vi "PIDMotor.vi"(0 "Motor Object":T5, 1 "Robot Configuration":T1={"wheel parameters"={"wheel radius"=0.05, "gear ratio"=1.0, "forward rotation direction"=0}, "wheel separation"=0.19, "Encoder Pulse Per Rev"=1856.0, "Update Period (sec)"=0.02, "Initial posture frame"=[0.0, 0.0, 0.0]} {"wheel parameters"."forward rotation direction" items=["Clockwise", "Counterclockwise"]}, 2 "calculated wheel states":T18[](array[typedef]), 3 "Wheel Velocity":T19) -> ()   [LabVIEW 2016]
uses:
  <vilib>/robotics/Steering/Wheel/Wheel State.ctl
  MotorObject.ctl
  <vilib>/myRIO/Instrument Drivers/Onboard IO/PWM/typedefs/PWM Reference.ctl
  <vilib>/myRIO/Common/Instrument Driver Framework/Utilities/typedefs/myRIO Generic Hardware Reference.ctl
  <vilib>/myRIO/Common/Instrument Driver Framework/Utilities/typedefs/Hardware Version Enum.ctl
  <vilib>/myRIO/Common/Instrument Driver Framework/Utilities/typedefs/myRIO v1.0 Reference.ctl
  <vilib>/myRIO/Common/Instrument Driver Framework/Utilities/typedefs/Generic FPGA Reference.ctl
  <vilib>/myRIO/Common/Instrument Driver Framework/myRIO v1.0/PWM/typedefs/PWM Channels Enum.ctl
  <vilib>/myRIO/Instrument Drivers/Onboard IO/PWM/typedefs/PWM Configuration.ctl
  <vilib>/myRIO/Instrument Drivers/Onboard IO/DIO/typedefs/DIO Reference.ctl
  <vilib>/myRIO/Common/Instrument Driver Framework/myRIO v1.0/DIO/typedefs/DIO Channels List.ctl
  <vilib>/myRIO/Common/Instrument Driver Framework/myRIO v1.0/DIO/typedefs/DIO Channels Enum.ctl
  <vilib>/myRIO/Instrument Drivers/Onboard IO/Encoder/typedefs/Encoder Reference.ctl
  <vilib>/myRIO/Common/Instrument Driver Framework/myRIO v1.0/Encoder/typedefs/Encoder Channels Enum.ctl
  Configurations.ctl
  <vilib>/robotics/Steering/Wheel/Wheel Parameters.ctl
  <vilib>/robotics/Steering/Wheel/Rotation Direction.ctl
  <vilib>/myRIO/Instrument Drivers/Onboard IO/PWM/vis/Set Duty Cycle and Frequency.vi
  <vilib>/myRIO/Common/Instrument Driver Framework/myRIO v1.0/DIO/vis/myRIO v1.0 Write DIO.vi
  <vilib>/myRIO/Common/Instrument Driver Framework/roboRIO v1.0/DIO/vis/roboRIO v1.0 Write DIO.vi
  <vilib>/Utility/error.llb/Error Cluster From Error Code.vi
  <vilib>/addons/control/pid/pid.llb/PID (DBL).vi
  <vilib>/myRIO/Common/Instrument Driver Framework/myRIO v1.0/PWM/vis/myRIO v1.0 Write PWM.vi
  <vilib>/myRIO/Common/Instrument Driver Framework/roboRIO v1.0/PWM/vis/roboRIO v1.0 Write PWM.vi
  <vilib>/addons/control/pid/NI_PID_pid.lvlib
  <vilib>/myRIO/Instrument Drivers/Onboard IO/PWM/PWM.lvlib
  <vilib>/myRIO/Instrument Drivers/Onboard IO/DIO/DIO.lvlib
  <vilib>/robotics/Steering/Wheel/NI_Robotics_Wheel.lvclass
  <vilib>/myRIO/Instrument Drivers/Onboard IO/Encoder/Encoder.lvlib
panel:
  out "DIR Right":bool
  in  "PID gains Motor Right":T4={"proportional gain (Kc)"=4.8, "integral time (Ti, min)"=0.01, "derivative time (Td, min)"=0.001} {"derivative time (Td, min)" format="%.3f"; "integral time (Ti, min)" format="%.3f"; "proportional gain (Kc)" format="%.3f"}
  out "PWM Signal Right":dbl
  out "PWM Signal Left":dbl
  in  "PID gains Motor Left":T4={"proportional gain (Kc)"=5.1, "integral time (Ti, min)"=0.01, "derivative time (Td, min)"=0.001} {"derivative time (Td, min)" format="%.3f"; "integral time (Ti, min)" format="%.3f"; "proportional gain (Kc)" format="%.3f"}
  out "DIR Left":bool
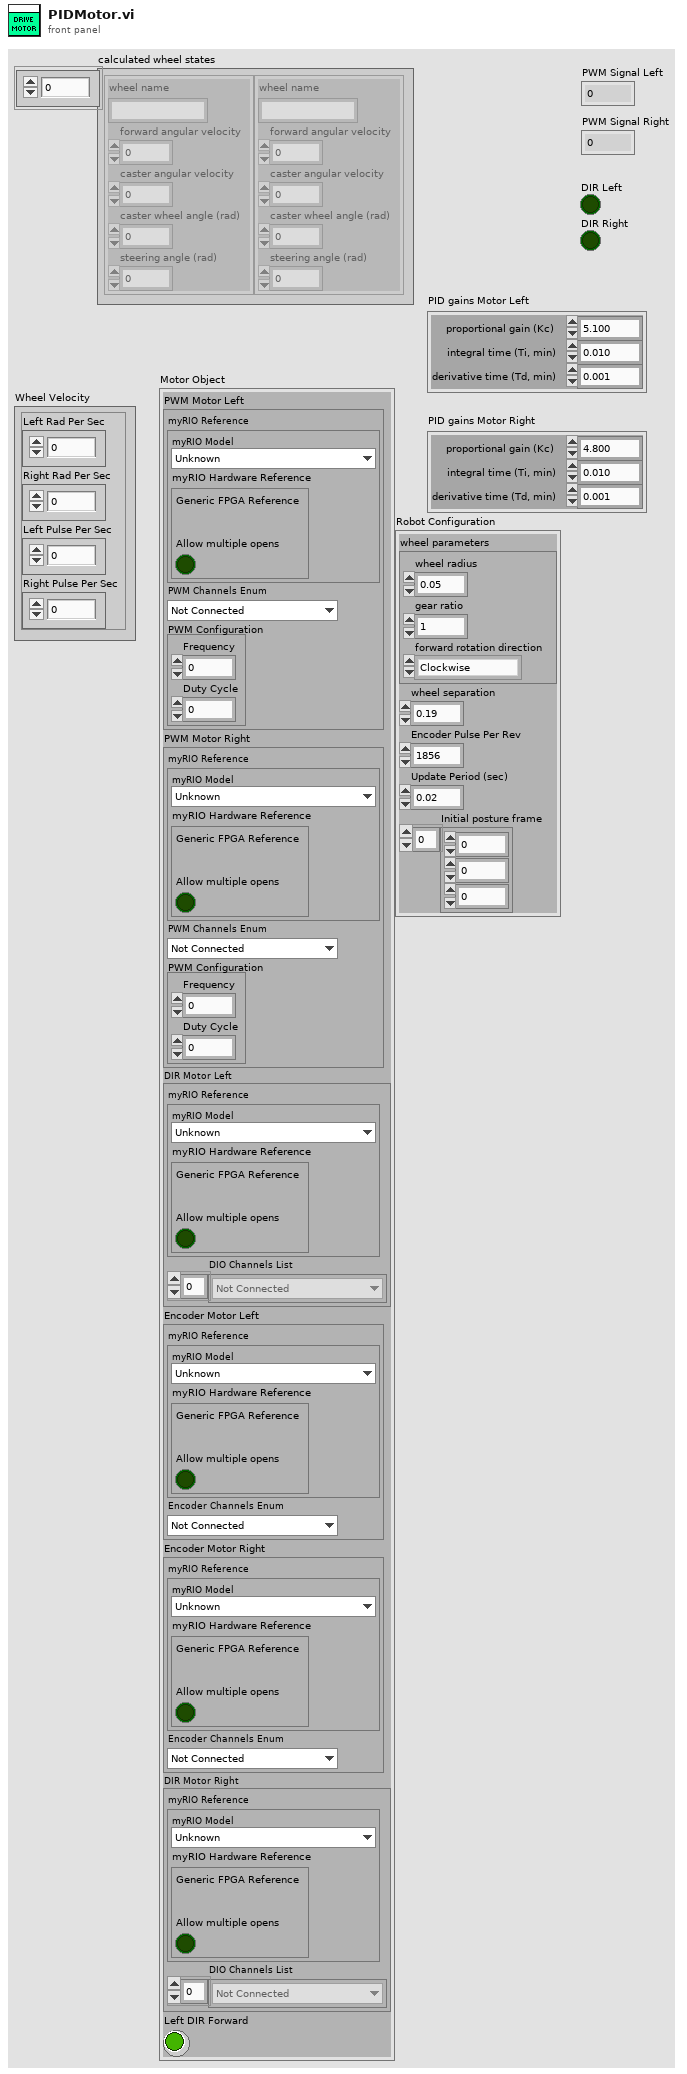
[diagram p1: front panel]
types:
  T1 = typedef "Configurations.ctl" = cluster{"wheel parameters":T2, "wheel separation":dbl, "Encoder Pulse Per Rev":dbl, "Update Period (sec)":dbl, "Initial posture frame":dbl[]}
  T2 = typedef "NI_Robotics_Wheel.lvclass/Wheel Parameters.ctl" = cluster{"wheel radius":dbl, "gear ratio":dbl, "forward rotation direction":T3}
  T3 = typedef "NI_Robotics_Wheel.lvclass/Rotation Direction.ctl" = u16
  T4 = cluster{"proportional gain (Kc)":dbl, "integral time (Ti, min)":dbl, "derivative time (Td, min)":dbl}
  T5 = typedef "MotorObject.ctl" = cluster{"PWM Motor Left":T6, "PWM Motor Right":T6, "DIR Motor Left":T13, "Encoder Motor Left":T16, "Encoder Motor Right":T16, "DIR Motor Right":T13, "Left DIR Forward":bool}
  T6 = typedef "PWM.lvlib/PWM Reference.ctl" = cluster{"myRIO Reference":T7, "PWM Channels Enum":T11, "PWM Configuration":T12}
  T7 = typedef "myRIO Generic Hardware Reference.ctl" = cluster{"myRIO Model":T8, "myRIO Hardware Reference":T9}
  T8 = typedef "Hardware Version Enum.ctl" = enum16{"Unknown", "myRIO-1900", "myRIO-1950", "roboRIO", "NI ELVIS RIO CM"}
  T9 = typedef "myRIO v1.0 Reference.ctl" = cluster{"Generic FPGA Reference":T10, "Allow multiple opens":bool}
  T10 = typedef "Generic FPGA Reference.ctl" = refnum<k20>
  T11 = typedef "PWM Channels Enum.ctl" = enum16{"Not Connected", "C/PWM0", "C/PWM1", "A/PWM0", "A/PWM1", "A/PWM2", "B/PWM0", "B/PWM1", "B/PWM2", "PWM/PWM0", "PWM/PWM1", "PWM/PWM2", "PWM/PWM3", "PWM/PWM4", "PWM/PWM5", "PWM/PWM6", "PWM/PWM7", "PWM/PWM8", "PWM/PWM9"}
  T12 = typedef "PWM.lvlib/PWM Configuration.ctl" = cluster{"Frequency":dbl, "Duty Cycle":dbl}
  T13 = typedef "DIO.lvlib/DIO Reference.ctl" = cluster{"myRIO Reference":T7, "DIO Channels List":T14}
  T14 = typedef "DIO Channels List.ctl" = T15[]
  T15 = typedef "DIO Channels Enum.ctl" = enum16{"Not Connected", "C/DIO0", "C/DIO1", "C/DIO2", "C/DIO3", "C/DIO4", "C/DIO5", "C/DIO6", "C/DIO7", "A/DIO0", "A/DIO1", "A/DIO2", "A/DIO3", "A/DIO4", "A/DIO5", "A/DIO6", "A/DIO7", "A/DIO8", "A/DIO9", "A/DIO10", "A/DIO11", "A/DIO12", "A/DIO13", "A/DIO14", "A/DIO15", "B/DIO0", "B/DIO1", "B/DIO2", "B/DIO3", "B/DIO4", "B/DIO5", "B/DIO6", "B/DIO7", "B/DIO8", "B/DIO9", "B/DIO10", "B/DIO11", "B/DIO12", "B/DIO13", "B/DIO14", "B/DIO15", "LED0", "LED1", "LED2", "LED3", "Button0", "DIO/DIO0", "DIO/DIO1", "DIO/DIO2", "DIO/DIO3", "DIO/DIO4", "DIO/DIO5", "DIO/DIO6", "DIO/DIO7", "DIO/DIO8", "DIO/DIO9", "SPI/CS0", "SPI/CS1", "SPI/CS2", "SPI/CS3", "LED RADIO (Green)", "LED RADIO (Red)", "LED COMM (Green)", "LED COMM (Red)", "LED MODE (Green)", "LED MODE (Red)"}
  T16 = typedef "Encoder.lvlib/Encoder Reference.ctl" = cluster{"myRIO Reference":T7, "Encoder Channels Enum":T17}
  T17 = typedef "Encoder Channels Enum.ctl" = enum16{"Not Connected", "C/ENC0", "C/ENC1", "A/ENC", "B/ENC", "DIO/ENC0", "DIO/ENC1", "DIO/ENC2", "DIO/ENC3", "DIO/ENC4"}
  T18 = typedef "NI_Robotics_Wheel.lvclass/Wheel State.ctl" = cluster{"wheel name":string, "forward angular velocity":dbl, "caster angular velocity":dbl, "caster wheel angle (rad)":dbl, "steering angle (rad)":dbl}
  T19 = cluster{"Left Rad Per Sec":dbl, "Right Rad Per Sec":dbl, "Left Pulse Per Sec":dbl, "Right Pulse Per Sec":dbl}
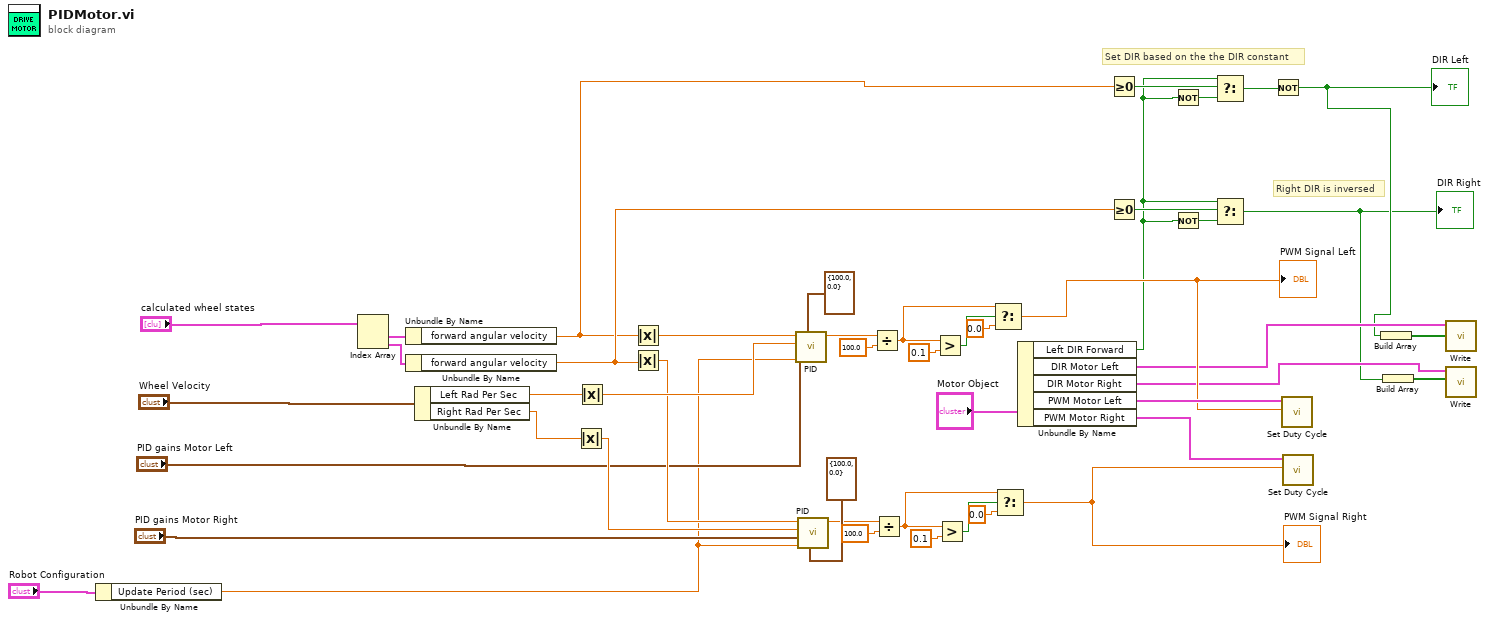
[diagram p0: block diagram]
diagram:
  # "Right DIR is inversed"
  # "Set DIR based on the the DIR constant"
  n1 = Unbundle By Name("Robot Configuration") -> ("Update Period (sec)"=w1:dbl)
  n2 = Index Array(array="calculated wheel states") -> (element #1=w36:T18, element #2=w37:T18)  [unwired: 2 in]
  n3 = Unbundle By Name(w36) -> ("forward angular velocity"=w5:dbl)
  n4 = Unbundle By Name(w37) -> ("forward angular velocity"=w6:dbl)
  n5 = Unbundle By Name("Wheel Velocity") -> ("Left Rad Per Sec"=w39:dbl, "Right Rad Per Sec"=w26:dbl)
  n6 = Absolute Value(x=w26) -> (abs(x)=w24:dbl)
  n7 = Absolute Value(x=w39) -> (abs(x)=w40:dbl)
  n8 = Absolute Value(x=w5) -> (abs(x)=w27:dbl)
  n9 = Absolute Value(x=w6) -> (abs(x)=w25:dbl)
  n10 = call-poly <vilib>:"PID.vi"("output range"=cluster{"output high":dbl, "output low":dbl} {"output high"=100.0, "output low"=0.0}, "dt (s)"=w1, "PID gains"="PID gains Motor Left", "process variable"=w40, "setpoint"=w27) -> ("output"=w47:dbl)  [unwired: 5 in, 1 out]
  n11 = call-poly <vilib>:"PID.vi"("output range"=cluster{"output high":dbl, "output low":dbl} {"output high"=100.0, "output low"=0.0}, "dt (s)"=w1, "PID gains"="PID gains Motor Right", "process variable"=w24, "setpoint"=w25) -> ("output"=w28:dbl)  [unwired: 5 in, 1 out]
  n12 = Divide(x=w47, y=100.0) -> (x/y=w45:dbl)
  n13 = Divide(x=w28, y=100.0) -> (x/y=w30:dbl)
  n14 = Greater?(x=w45, y=0.1) -> (0:w44:bool)
  n15 = Greater?(x=w30, y=0.1) -> (0:w31:bool)
  n16 = Select(t=w45, s=w44, f=0.0) -> (s? t:f=w19:dbl)
  "PWM Signal Left" <- w19
  n17 = Select(t=w30, s=w31, f=0.0) -> (s? t:f=w18:dbl)
  "PWM Signal Right" <- w18
  n18 = Unbundle By Name("Motor Object") -> ("Left DIR Forward"=w13:bool, "DIR Motor Left"=w12:T13, "DIR Motor Right"=w11:T13, "PWM Motor Left"=w21:T6, "PWM Motor Right"=w20:T6)
  n19 = Greater Or Equal To 0?(x=w5) -> (x >= 0?=w14:bool)
  n20 = Greater Or Equal To 0?(x=w6) -> (x >= 0?=w17:bool)
  n21 = Not(x=w13) -> (.not. x?=w15:bool)
  n22 = Not(x=w13) -> (.not. x?=w16:bool)
  n23 = Select(t=w13, s=w14, f=w15) -> (s? t:f=w10:bool)
  n24 = Select(t=w13, s=w17, f=w16) -> (s? t:f=w3:bool)
  "DIR Right" <- w3
  n25 = Not(x=w10) -> (.not. x?=w4:bool)
  "DIR Left" <- w4
  n26 = call <vilib>:"Set Duty Cycle.vi"("Duty Cycle"=w19, "PWM Ref In"=w21) -> ()  [unwired: 7 in, 2 out]
  n27 = call <vilib>:"Set Duty Cycle.vi"("Duty Cycle"=w18, "PWM Ref In"=w20) -> ()  [unwired: 7 in, 2 out]
  n28 = Build Array(w4) -> (w9:bool[])
  n29 = Build Array(w3) -> (w8:bool[])
  n30 = call <vilib>:"Write.vi"("Values"=w9, "DIO Ref In"=w12) -> ()  [unwired: 7 in, 2 out]
  n31 = call <vilib>:"Write.vi"("Values"=w8, "DIO Ref In"=w11) -> ()  [unwired: 7 in, 2 out]
